vi "LCM of P(x) and Q(x) (DBL).vi"(8 "algorithm":u16(ring) items=["Euclidean", "Approximate GCD"], 9 "tolerance":dbl=1e-07 format="%#.6g", 10 "Q(x)":dbl[](array[numeric]) format="%#.6g", 11 "P(x)":dbl[](array[numeric]) format="%#.6g") -> (0 "error":i32, 3 "Least Common Multiple":dbl[](array[numeric]) format="%#.6g")   [LabVIEW 2024, in "NI_AALPro.lvlib"]
doc: "<p>Computes the least common multiple of two polynomials <strong>P(x)</strong> and <strong>Q(x)</strong> with the <strong>tolerance</strong> you specify. The data types you wire to the <strong>P(x)</strong> and <strong>Q(x)</strong> inputs determine the polymorphic instance to use.</p>"
uses:
  NI_AALPro.lvlib
  Polynomial GCD Pair (DBL).vi
  Remove Zero Coefficients (DBL).vi
  Multiply Polynomials (DBL).vi
  GCD of P(x) and Q(x) (DBL).vi
  Divide Polynomials (DBL).vi
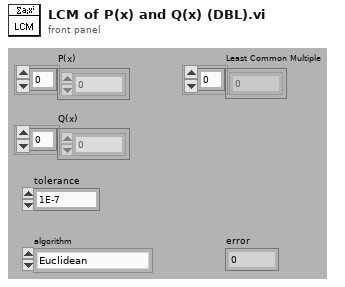
[diagram p1: front panel]
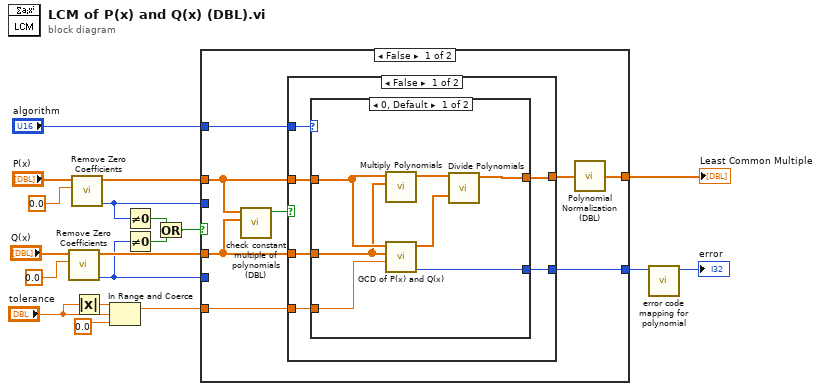
[diagram p0: block diagram]
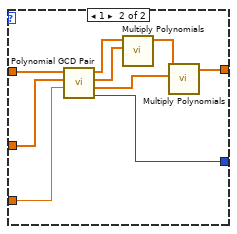
[diagram p2: hidden frame]
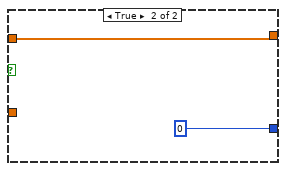
[diagram p3: hidden frame]
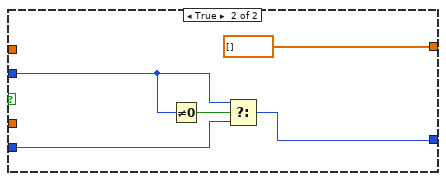
[diagram p4: hidden frame]
diagram:
  n1 = call-poly "Remove Zero Coefficients.vi"("threshold"=0.0, "P(x) In"="Q(x)") -> ("error"=w5:i32, "P(x) Out"=w10:dbl[])  [unwired: 7 in, 1 out]
  n2 = call-poly "Remove Zero Coefficients.vi"("threshold"=0.0, "P(x) In"="P(x)") -> ("error"=w6:i32, "P(x) Out"=w9:dbl[])  [unwired: 7 in, 1 out]
  n3 = Absolute Value(x="tolerance") -> (abs(x)=w17:dbl)
  n4 = In Range and Coerce(upper limit=w17, x="tolerance", lower limit=0.0) -> (coerced(x)=w16:dbl)  [unwired: 1 out]
  n5 = Not Equal To 0?(x=w6) -> (x != 0?=w4:bool)
  n6 = Not Equal To 0?(x=w5) -> (x != 0?=w3:bool)
  n7 = Or(x=w4, y=w3) -> (x .or. y?=w2:bool)
  n8 = case shown="False" w2 {
    tunnel: w9 -> [w25 _]
    tunnel: w10 -> [w24 _]
    tunnel: [w23 dbl[] [] ("BDL")] -> w19
    tunnel: w16 -> [w27 _]
    tunnel: [w26 w52] -> w8
    tunnel: w6 -> [_ w54]
    tunnel: w5 -> [_ w53]
    tunnel: "algorithm" -> [w20 _]
    frame False {
      n9 = call "check constant multiple of polynomials (DBL).vi"("Q(x)"=w24, "P(x)"=w25) -> ("constant multiple?"=w22:bool)  [unwired: 9 in]
      n10 = case shown="False" w22 {
        tunnel: [w29 w51] -> w21
        tunnel: w27 -> [w33 _]
        tunnel: [w32 0 ("error")] -> w26
        tunnel: w25 -> [w31 w51]
        tunnel: w24 -> [w30 _]
        tunnel: w20 -> [w28 _]
        frame False {
          n11 = case shown="0, Default" w28 {
            tunnel: w33 -> [w39 w47]
            tunnel: [w38 w41] -> w32
            tunnel: w31 -> [w36 w49]
            tunnel: w30 -> [w35 w48]
            tunnel: [w34 w44] -> w29
            frame 0, Default {
              n12 = call-poly "Multiply Polynomials.vi"("Q(x)"=w35, "P(x)"=w36) -> ("P(x)*Q(x)"=w40:dbl[])  [unwired: 8 in, 1 out]
              n13 = call-poly "GCD of P(x) and Q(x).vi"("tolerance"=w39, "Q(x)"=w35, "P(x)"=w36) -> ("error"=w38:i32, "Greatest Common Divisor"=w37:dbl[])  [unwired: 7 in]
              n14 = call-poly "Divide Polynomials.vi"("Q(x)"=w37, "P(x)"=w40) -> ("P(x)/Q(x)"=w34:dbl[])  [unwired: 7 in, 2 out]
            }
            frame 1 {
              n15 = call-poly "Polynomial GCD Pair.vi"("tolerance"=w47, "Q(x)"=w48, "P(x)"=w49) -> ("error"=w41:i32, "Co-factor of Q(x)"=w42:dbl[], "Co-factor of P(x)"=w45:dbl[], "Greatest Common Divisor"=w46:dbl[])  [unwired: 5 in]
              n16 = call-poly "Multiply Polynomials.vi"("Q(x)"=w45, "P(x)"=w46) -> ("P(x)*Q(x)"=w43:dbl[])  [unwired: 8 in, 1 out]
              n17 = call-poly "Multiply Polynomials.vi"("Q(x)"=w42, "P(x)"=w43) -> ("P(x)*Q(x)"=w44:dbl[])  [unwired: 8 in, 1 out]
            }
          }
        }
        frame True {
        }
      }
      n18 = call "Polynomial Normalization (DBL).vi"("polynomial"=w21) -> ("normalized polynomial"=w23:dbl[])
    }
    frame True {
      n19 = Not Equal To 0?(x=w54) -> (x != 0?=w55:bool)
      n20 = Select(t=w54, s=w55, f=w53) -> (s? t:f=w52:i32)
    }
  }
  "Least Common Multiple" <- w19
  n21 = call "error code mapping for polynomial.vi"("error in"=w8) -> ("error out"=→"error":i32)  [unwired: 10 in]
